vi "Create.vi"(8 "error in (no error)":errorcluster, 11 "Path":path) -> (0 "error out":errorcluster, 3 "Reader":refnum<class "Reader.lvclass">)   [LabVIEW 2020, in "video_io.lvlib" / "Reader.lvclass"]
uses:
  Reader.lvclass
  Reader.lvclass/Reader.ctl
  common/bin/gartoolkit_videoio_32-1.dll
  common/common.lvlib
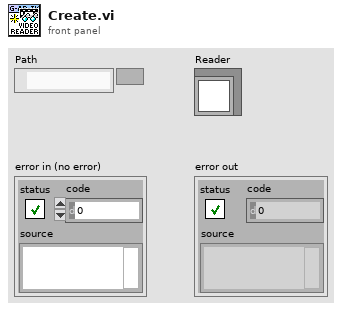
[diagram p1: front panel]
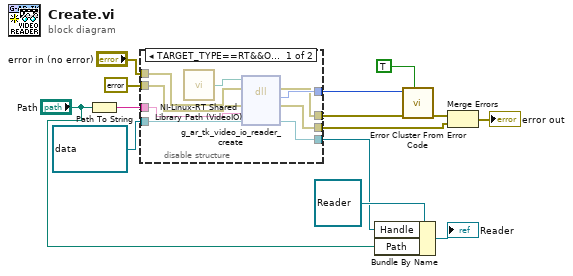
[diagram p0: block diagram]
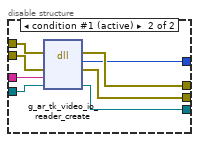
[diagram p2: hidden frame]
diagram:
  n1 = Path To String(path="Path") -> (string=w5:string)
  n2 = disable-structure shown="TARGET_TYPE==RT&&OS==Linux" {
    disable-tunnel: "error in (no error)" -> [w23 w31]
    disable-tunnel: errorcluster {"status"=FALSE, "code"=0, "source"=""} ("error constant") -> [w22 w30]
    disable-tunnel: w5 -> [w21 w24]
    disable-tunnel: refnum<data-value> refnum ("EDVR") -> [w20 w29]
    disable-tunnel: [w16 w28] -> w10
    disable-tunnel: [w18 w27] -> w9
    disable-tunnel: [w17 w26] -> w3
    disable-tunnel: [w15 w25] -> w7
    frame condition #0 {
      n3 = call "NI-Linux-RT Shared Library Path (VideoIO).vi"() -> ("Path"=w19:path)
      n4 = dll-call lib="?" fn="g_ar_tk_video_io_reader_create" ("g_ar_toolkit.*.*:g_ar_tk_capture_context_create")(path in=w19, error in=w23, "error_cluster"=w22, "Path"=w21, "Handle"=w20) -> (error out=w16:errorcluster, "return type"=w18:i32, "error_cluster"=w15:errorcluster, "Handle"=w17:refnum<data-value>)  [unwired: 2 in, 1 out]
    }
    frame condition #1 (active) {
      n5 = dll-call lib="C:/serenial/lib/g-augmented-reality-toolkit/LabVIEW/common/bin/gartoolkit_videoio_*-1.*" fn="g_ar_tk_video_io_reader_create" ("g_ar_toolkit.*.*:g_ar_tk_capture_context_create")(error in=w31, "error_cluster"=w30, "Path"=w24, "Handle"=w29) -> (error out=w28:errorcluster, "return type"=w27:i32, "error_cluster"=w25:errorcluster, "Handle"=w26:refnum<data-value>)  [unwired: 3 in, 1 out]
    }
  }
  n6 = Bundle By Name(cluster=refnum<class "Reader.lvclass"> refnum ("video_io.lvlib:Reader.lvclass"), "Handle"=w3, "Path"="Path") -> (→"Reader":refnum<class "Reader.lvclass">)
  n7 = call <vilib>:"Error Cluster From Error Code.vi"("show call chain? (False)"=TRUE, "error in (no error)"=w10, "error code (0)"=w9) -> ("error out"=w14:errorcluster)  [unwired: 6 in]
  n8 = Merge Errors(w14, w7) -> (→"error out":errorcluster)
